vi "GT_LnXYG0.vi"(5 "X":i32, 6 "synAcc":dbl, 7 "Y":i32, 8 "synVel":dbl, 9 "fifo":i16, 10 "crd":i16, 11 "rtn_In":cluster{"rtn":i16, "Func":string}) -> (1 "fifo out":i16, 2 "crd out":i16, 3 "rtn_Out":cluster{"rtn":i16, "Func":string})   [LabVIEW 2014]
uses:
  VC6/gts.dll
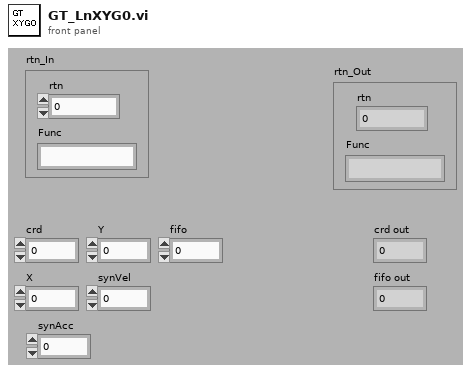
[diagram p1: front panel]
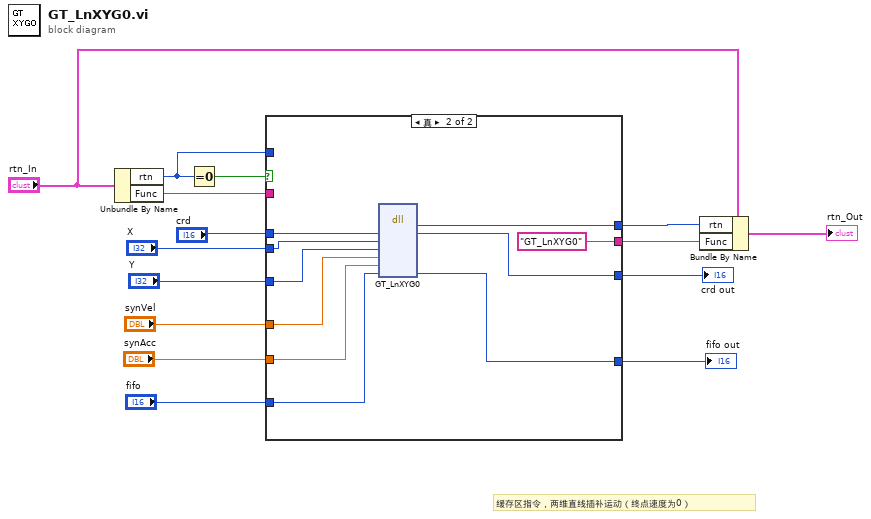
[diagram p0: block diagram]
diagram:
  # "缓存区指令，两维直线插补运动（终点速度为0）"
  n1 = Unbundle By Name("rtn_In") -> ("rtn"=w2:i16, "Func"=w1:string)
  n2 = Equal To 0?(x=w2) -> (x = 0?=w15:bool)
  n3 = case shown="真" w15 {
    tunnel: [w18 "GT_LnXYG0" ("Func")] -> w12
    tunnel: [w19 w28] -> w11
    tunnel: "crd" -> [w17 w27]
    tunnel: [w17 w26] -> w9
    tunnel: "X" -> [_ w25]
    tunnel: "Y" -> [_ w24]
    tunnel: "synVel" -> [_ w23]
    tunnel: "synAcc" -> [_ w22]
    tunnel: "fifo" -> [w16 w21]
    tunnel: [w16 w20] -> w3
    tunnel: w2 -> [w19 _]
    tunnel: w1 -> [w18 _]
    frame False {
    }
    frame True {
      n4 = dll-call lib="PTH2Fabs DNewGTS AC-800LWin7版源程序-20170926gts85VC6gts.dll" fn="GT_LnXYG0"("crd"=w27, "X"=w25, "Y"=w24, "synVel"=w23, "synAcc"=w22, "fifo"=w21) -> ("rtn"=w28:i16, "crd"=w26:i16, "fifo"=w20:i16)  [unwired: 7 in, 2 out]
    }
  }
  "crd out" <- w9
  "fifo out" <- w3
  n5 = Bundle By Name(cluster="rtn_In", "rtn"=w11, "Func"=w12) -> (→"rtn_Out":cluster{"rtn":i16, "Func":string})
